vi "add_float32.vi"   [LabVIEW 2012]
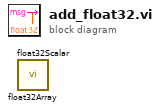
[diagram p0: block diagram]
diagram:
  n1 = call "float32Array.vi"() -> ()  [unwired: 5 in, 1 out]
  n2 = call "float32Scalar.vi"() -> ()  [unwired: 5 in, 1 out]
